vi "Test SFOAE Circular Buffer.vi"() -> ()   [LabVIEW 2015]
uses:
  Typedefs/SFOAE-Stimulus Parameters.ctl
  Typedefs/SFOAE-Sweep Params.ctl
  Typedefs/SFOAE-AO Runtime Data.ctl
panel:
  in  "Cal Folder":path=path "C:/Experiment VIs/Cochlear Function Test Suite/LV Source/SFOAE VIs/Test VIs"
  out "Waveform Graph":dbl[][](graph)
  in  "Fs (Hz)":dbl=100000.0
  in  "SFOAE Stim":T1={"Ear"=enum."Right", "Sweep"={"Type"=enum."Linear", "Fmin (kHz)"=4.0, "Fmax (kHz)"=8.0, "Rate"=2.0, "Ramp (ms)"=5.0, "Drain (ms)"=20.0}, "Suppressor"={"Delta"=50.0, "Ratio"=0.0, "Use ratio"=FALSE}, "Concurrent"={"Nsweeps"=1, "Overlap"=0.0}, "Ls (dB SPL)"=50.0, "Lp (dB SPL)"={"Min"=50.0, "Max"=50.0, "Step"=5.0}}
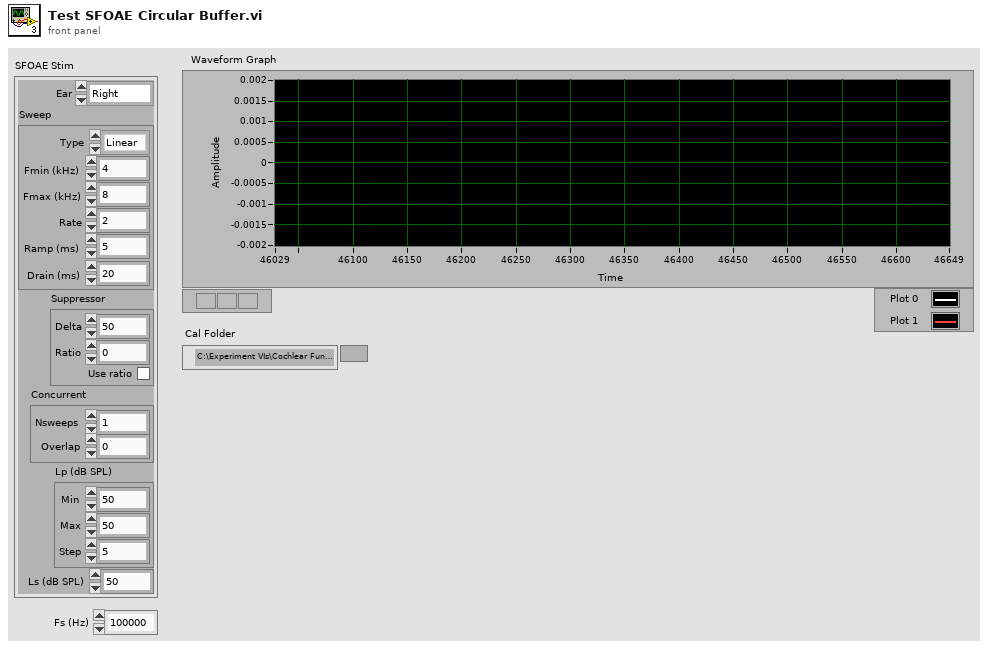
[diagram p1: front panel]
types:
  T1 = typedef "SFOAE-Stimulus Parameters.ctl" = cluster{"Ear":enum16{"Right", "Left"}, "Sweep":T2, "Suppressor":cluster{"Delta":dbl, "Ratio":dbl, "Use ratio":bool}, "Concurrent":cluster{"Nsweeps":i32, "Overlap":dbl}, "Ls (dB SPL)":dbl, "Lp (dB SPL)":cluster{"Min":dbl, "Max":dbl, "Step":dbl}}
  T2 = typedef "SFOAE-Sweep Params.ctl" = cluster{"Type":enum16{"Linear", "Log"}, "Fmin (kHz)":dbl, "Fmax (kHz)":dbl, "Rate":dbl, "Ramp (ms)":dbl, "Drain (ms)":dbl}
  T3 = typedef "SFOAE-AO Runtime Data.ctl" = cluster{"AO":i32[], "Frame size":i32, "CurPos":i32, "probe":dbl[], "suppressor":dbl[], "CurStim":i32, "StimLen":i32}
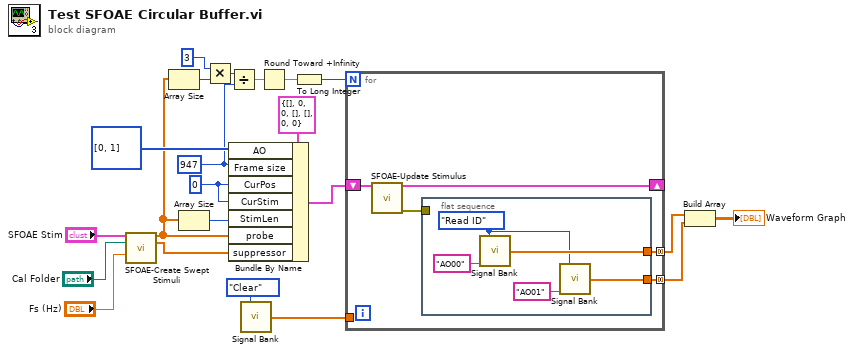
[diagram p0: block diagram]
diagram:
  w10 = 947 ("Frame size")
  w6 = 0 ("CurPos")
  n1 = call "SFOAE-Create Swept Stimuli.vi"("SFOAE Stim"="SFOAE Stim", "Data Folder"="Cal Folder", "Fs (Hz)"="Fs (Hz)") -> ("probe"=w5:dbl[], "suppressor"=w18:dbl[])  [unwired: 8 in, 3 out]
  n2 = Array Size(array=w5) -> (size(s)=w14:i32)
  n3 = Array Size(array=w5) -> (size(s)=w4:i32)
  n4 = Multiply(x=3, y=w14) -> (x*y=w8:i32)
  n5 = Divide(x=w8, y=w10) -> (x/y=w12:dbl)
  n6 = Bundle By Name(cluster=T3 {"AO"=[], "Frame size"=0, "CurPos"=0, "probe"=[], "suppressor"=[], "CurStim"=0, "StimLen"=0} ("AO Runtime"), "AO"=i32[] [0, 1], "Frame size"=w10, "CurPos"=w6, "CurStim"=w6, "StimLen"=w4, "probe"=w5, "suppressor"=w18) -> (w17:T3)
  n7 = call "Signal Bank.vi"("Action"=enum16{"Add", "Replace ID", "Read ID", "Clear"}."Clear") -> ("1D Data Out"=w15:dbl[])  [unwired: 13 in, 1 out]
  n8 = Round Toward +Infinity(x=w12) -> (ceil(x): smallest int >= x=w11:dbl)
  n9 = To Long Integer(number=w11) -> (32bit integer=w9:i32)
  n10 = for {
    N: w9 -> [_]
    shift-right: [w26] -> _
    shift-left: w17 -> [w27]
    tunnel: [w25] -> w3 mode=concatenating
    tunnel: w15 -> [_]
    tunnel: [w23] -> w2 mode=concatenating
    n11 = call "SFOAE-Update Stimulus.vi"("AO Runtime in"=w27) -> ("AO Runtime out"=w26:T3, "error out"=w24:errorcluster)  [unwired: 13 in]
    n12 = flat-sequence {
      tunnel: [w31] -> w25
      tunnel: w24 -> [_]
      tunnel: [w28] -> w23
      frame #0 {
        w29 = enum16{"Add", "Replace ID", "Read ID", "Clear"}."Read ID" ("Action")
        n13 = call "Signal Bank.vi"("Action"=w29, "ID"="AO00") -> ("1D Data Out"=w31:dbl[])  [unwired: 12 in, 1 out]
        n14 = call "Signal Bank.vi"("Action"=w29, "ID"="AO01") -> ("1D Data Out"=w28:dbl[])  [unwired: 12 in, 1 out]
      }
    }
  }
  n15 = Build Array(w3, w2) -> (→"Waveform Graph":dbl[][])
